vi "Area Scoring.vi"(10 "Convex Hull Area":dbl, 11 "Area":dbl) -> (3 "Score":dbl)   [LabVIEW 2017]
doc: "Calculate a score based on area and convex hull area. Convex hull area fills holes and convex areas of the shape. It is equivalent to putting a rubber band around the shape and computing the area enclosed by the band."
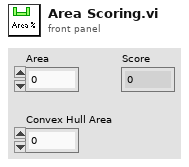
[diagram p1: front panel]
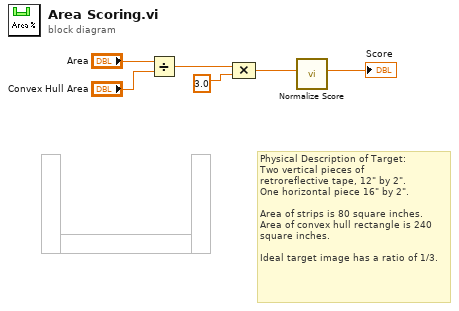
[diagram p0: block diagram]
diagram:
  # "Physical Description of Target:\nTwo vertical pieces of\nretroreflective tape, 12\" by 2\".\nOne horizontal piece 16\" by 2\".\n\nArea of strips is 80 square inches.\nArea of convex hull rectangle is 240\nsquare inches.\n\nIdeal target image has a ratio of 1/3."
  n1 = Divide(x="Area", y="Convex Hull Area") -> (x/y=w4:dbl)
  n2 = Compound Arithmetic op=MULTIPLY(w4, 3.0 ("length")) -> (w2:dbl)
  n3 = call "Normalize Score.vi"("Value"=w2) -> ("Score"=→"Score":dbl)  [unwired: 10 in]
